vi "20.2.-Data Socket Bidireccional 2.vi"() -> ()   [LabVIEW 2017]
panel:
  out "error out":errorcluster
  out "Slide":u8(slide) scale=0.0..10.0
  in  "Boolean":bool
  in  "stop":bool
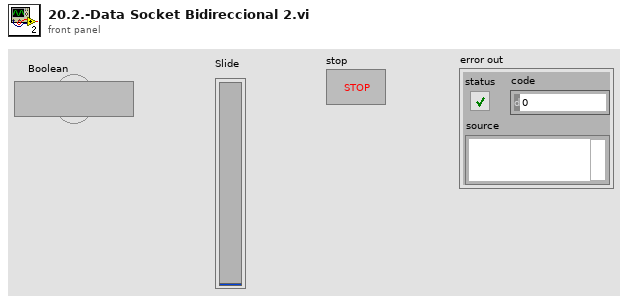
[diagram p1: front panel]
types:
  T1 = enum16{"Read", "Write", "ReadWrite", "BufferedRead", "BufferedReadWrite"}
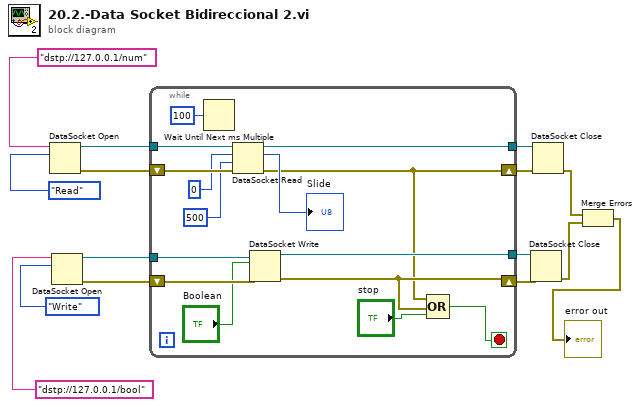
[diagram p0: block diagram]
diagram:
  n1 = DataSocket Open(10:T1."Read" ("mode"), 11:"dstp://127.0.0.1/num" ("URL")) -> (0:w9:errorcluster, 3:w11:refnum<k13>)  [unwired: 2 in]
  n2 = DataSocket Open(10:T1."Write" ("mode"), 11:"dstp://127.0.0.1/bool" ("URL")) -> (0:w8:errorcluster, 3:w10:refnum<k13>)  [unwired: 2 in]
  n3 = while {
    tunnel: w11 -> [w30]
    tunnel: w10 -> [w28]
    shift-right: [w17] -> w6
    shift-left: w9 -> [w29]
    shift-right: [w18] -> w4
    shift-left: w8 -> [w27]
    tunnel: [w21] -> w7
    tunnel: [w20] -> w5
    stop <- w16 stop-if-true
    n4 = Wait Until Next ms Multiple(millisecond multiple=u32 100) -> ()  [unwired: 1 out]
    n5 = DataSocket Read(8:w29, 9:500 ("ms timeout (0)"), 10:0, 11:w30) -> (0:w17:errorcluster, 2:→"Slide":i32, 3:w21:refnum<k13>)  [unwired: 1 in, 4 out]
    n6 = DataSocket Write(8:w27, 10:"Boolean", 11:w28) -> (0:w18:errorcluster, 3:w20:refnum<k13>)  [unwired: 1 in, 1 out]
    n7 = Compound Arithmetic op=OR(w17, w18, "stop") -> (w16:bool)
  }
  n8 = DataSocket Close(8:w4, 11:w5) -> (0:w2:errorcluster)  [unwired: 1 in, 1 out]
  n9 = DataSocket Close(8:w6, 11:w7) -> (0:w3:errorcluster)  [unwired: 1 in, 1 out]
  n10 = Merge Errors(w3, w2) -> (→"error out":errorcluster)
